vi "VoltageFailure.vi"(0 "Voltage_Configurations":T1={"Maximum(V)"=5.0, "Minimum(V)"=3.0, "Resolution(V)"=0.01} {"Resolution(V)" min=0.01 max=0.01; "Minimum(V)" min=3.0 max=3.0; "Maximum(V)" min=3.0 max=5.0 step=0.01}) -> (4 "Voltage_Failure_Point(V)":dbl)   [LabVIEW 2020]
doc: "This VI finds the lowest failure point of a device in the voltage range of 3-5V at a resolution of 10mV\nfor the varying model"
uses:
  Typedefs/VoltageInput.ctl
panel:
  out "Time(s)":dbl
  # "Voltage Failing Point"
  # "This program finds the lowest value at which the device fails\nto function asper the functionality."
  # "OUTPUT"
  # "INPUT"
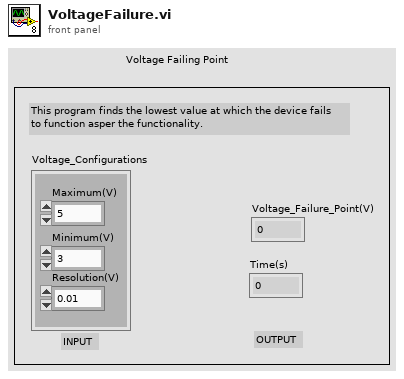
[diagram p1: front panel]
types:
  T1 = typedef "VoltageInput.ctl" = cluster{"Maximum(V)":dbl, "Minimum(V)":dbl, "Resolution(V)":dbl}
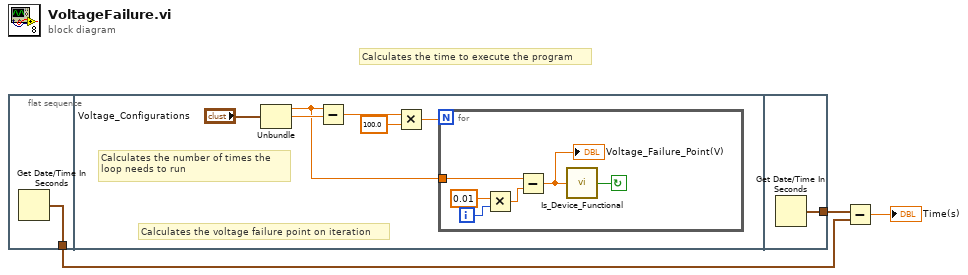
[diagram p0: block diagram]
diagram:
  # "Calculates the time to execute the program"
  n1 = flat-sequence {
    tunnel: [w4] -> w2
    tunnel: [w17] -> w3
    frame #0 {
      n2 = Get Date/Time In Seconds() -> (seconds since 1Jan1904=w4:timestamp)
    }
    frame #1 {
      # "Calculates the voltage failure point on iteration"
      # "Calculates the number of times the \nloop needs to run"
      n3 = Unbundle("Voltage_Configurations") -> ("Maximum(V)"=w5:dbl, "Minimum(V)"=w6:dbl)  [unwired: 1 out]
      n4 = Subtract(x=w5, y=w6) -> (x-y=w9:dbl)
      n5 = Multiply(x=w9, y=100.0) -> (x*y=w7:dbl)
      n6 = for {
        N: w7 -> [_]
        tunnel: w5 -> [w11]
        i -> [w13]
        stop <- w15 continue-if-true
        n7 = Multiply(x=0.01, y=w13) -> (x*y=w12:dbl)
        n8 = Subtract(x=w11, y=w12) -> (x-y=w16:dbl)
        "Voltage_Failure_Point(V)" <- w16
        n9 = call "Is_Device_Functional.vi"("Operating_Voltage(V)"=w16) -> ("Device_Functional"=w15:bool)  [unwired: 14 in]
      }
    }
    frame #2 {
      n10 = Get Date/Time In Seconds() -> (seconds since 1Jan1904=w17:timestamp)
    }
  }
  n11 = Subtract(x=w3, y=w2) -> (x-y=→"Time(s)":dbl)
